vi "Configure.vi"(8 "error in (no error)":errorcluster, 11 "ImageStack in":refnum<class "ImageStack.lvclass">) -> (0 "error out":errorcluster, 2 "cancelled?":bool, 3 "ImageStack out":refnum<class "ImageStack.lvclass">)   [LabVIEW 2012, in "ImageStack.lvclass"]
doc: "The configure method configures the details for the RabbitMQ connection. \n\nIn the derived class, make a call to the parent for setting these parameters."
uses:
  ImageStack.lvclass
  <vilib>/Utility/miscctls.llb/LVPointTypeDef.ctl
  ImageStack.lvclass/ImageStack.ctl
  <vilib>/Distrio/Murmex/Murmex/Murmex.lvclass
panel:
  in  "AOTF component name":string
  in  "button:cancel":bool
  in  "button:configure murmex":bool
  in  "button:ok":bool
  in  "Stages component name":string
  in  "Camera component name":string
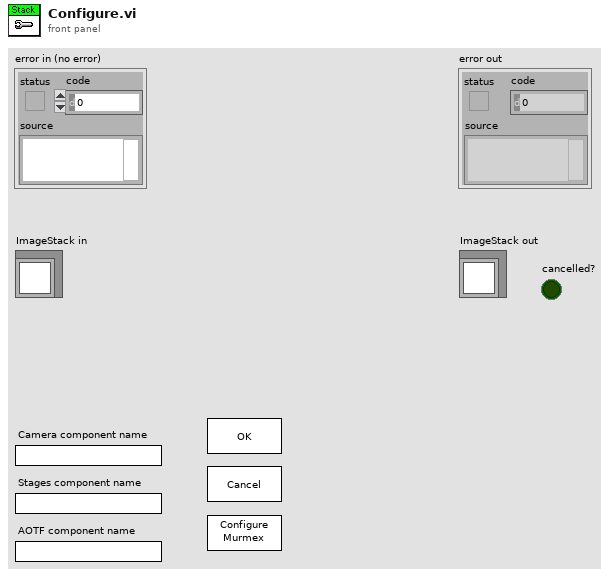
[diagram p1: front panel]
types:
  T1 = typedef "LVPointTypeDef.ctl" = cluster{"Horizontal":i16, "Vertical":i16}
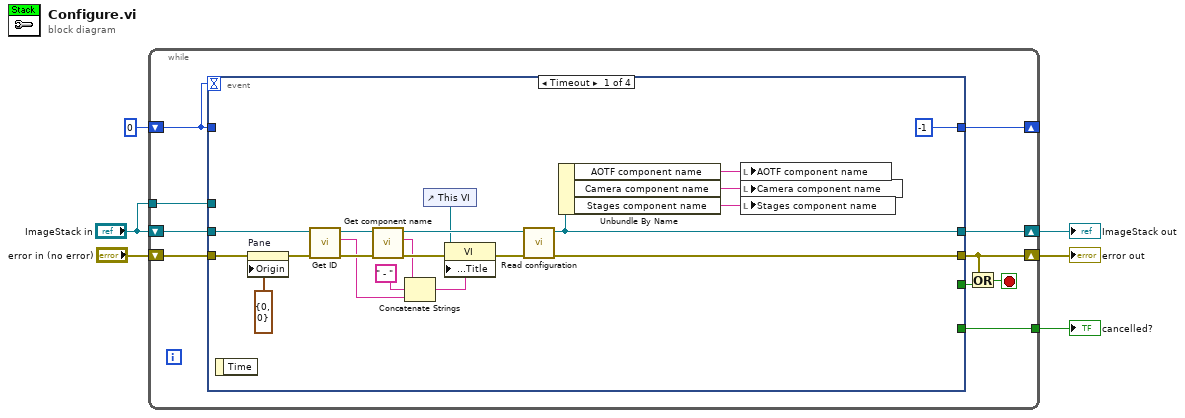
[diagram p0: block diagram]
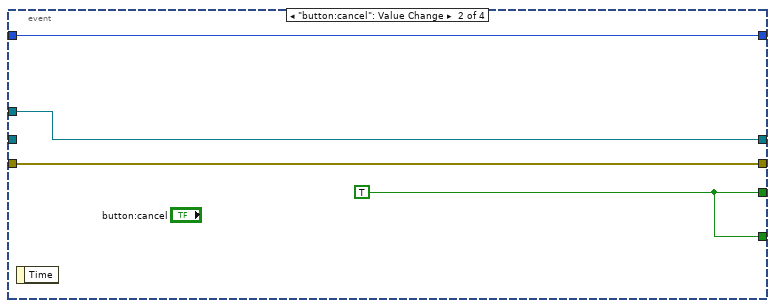
[diagram p2: hidden frame]
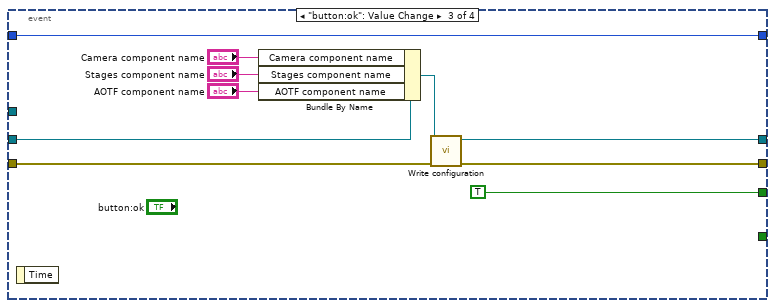
[diagram p3: hidden frame]
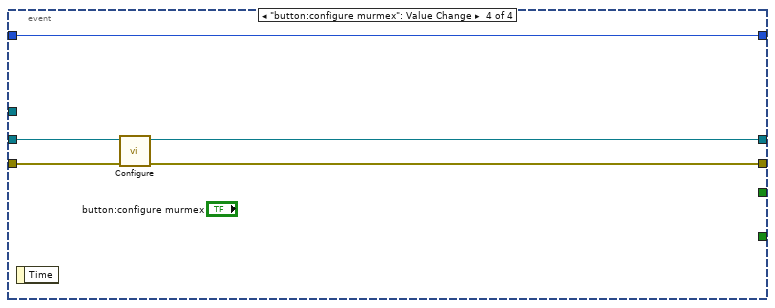
[diagram p4: hidden frame]
diagram:
  n1 = while {
    shift-right: [w11] -> w1
    shift-left: "ImageStack in" -> [w12]
    shift-right: [w13] -> w2
    shift-left: "error in (no error)" -> [w15]
    shift-right: [w16] -> _
    shift-left: 0 -> [w8]
    tunnel: "ImageStack in" -> [w9]
    tunnel: [w7] -> w3
    stop <- w14 stop-if-true
    n2 = event shown="[0] Timeout" {
      selector: _ -> [_ _ _ _]
      dyn-events: _ -> [_ _ _ _]
      timeout: w8 -> [_ _ _ _]
      tunnel: [-1 w38 w42 w51] -> w16
      tunnel: w15 -> [w34 w40 w46 w54]
      tunnel: [w35 w40 w44 w52] -> w13
      tunnel: w12 -> [w31 _ w50 w55]
      tunnel: [w20 w39 w45 w53] -> w11
      tunnel: [_ w37 TRUE _] -> w10
      tunnel: w9 -> [_ w39 _ _]
      tunnel: w8 -> [_ w38 w42 w51]
      tunnel: [_ w37 _ _] -> w7
      event Timeout {
        n3 = event-data() -> ()  [unwired: 1 in, 1 out]
        n4 = property on="Pane" class="Pane"(error in=w34, "Origin"=T1 {"Horizontal"=0, "Vertical"=0}) -> (error out=w32:errorcluster)  [unwired: 1 in, 1 out]
        n5 = call <vilib>:"Get ID.vi"("error in (no error)"=w32, "Murmex in"=w31) -> ("error out"=w29:errorcluster, "component id"=w25:string, "Murmex out"=w30:refnum<class "ImageStack.lvclass">)  [unwired: 7 in]
        n6 = call <vilib>:"Get component name.vi"("error in (no error)"=w29, "Murmex in"=w30) -> ("error out"=w28:errorcluster, "component name"=w26:string, "Murmex out"=w27:refnum<class "ImageStack.lvclass">)  [unwired: 7 in]
        n7 = Concatenate Strings(w26, " - " ("element"), w25) -> (w21:string)
        n8 = control-ref of="This VI"() -> (w22:refnum<vi>)
        n9 = property class="VI"(reference=w22, error in=w28, "Front Panel.Title"=w21) -> (error out=w23:errorcluster)  [unwired: 1 out]
        n10 = call <vilib>:"Read configuration.vi"("error in (no error)"=w23, "Murmex in"=w27) -> ("error out"=w35:errorcluster, "Murmex out"=w20:refnum<class "ImageStack.lvclass">)  [unwired: 7 in, 1 out]
        n11 = Unbundle By Name(w20) -> ("AOTF component name"=w17:string, "Camera component name"=w19:string, "Stages component name"=w18:string)
        n12 = local write "AOTF component name"(w17) -> ()
        n13 = local write "Camera component name"(w19) -> ()
        n14 = local write "Stages component name"(w18) -> ()
      }
      event "button:cancel": Value Change {
        w37 = TRUE
        n15 = event-data() -> ()  [unwired: 1 in, 1 out]
      }
      event "button:ok": Value Change {
        n16 = event-data() -> ()  [unwired: 1 in, 1 out]
        n17 = Bundle By Name(cluster=w50, "Camera component name"="Camera component name", "Stages component name"="Stages component name", "AOTF component name"="AOTF component name") -> (w49:refnum<class "ImageStack.lvclass">)
        n18 = call <vilib>:"Write configuration.vi"("error in (no error)"=w46, "Murmex in"=w49) -> ("error out"=w44:errorcluster, "Murmex out"=w45:refnum<class "ImageStack.lvclass">)  [unwired: 8 in]
      }
      event "button:configure murmex": Value Change {
        n19 = event-data() -> ()  [unwired: 1 in, 1 out]
        n20 = call-parent "Configure.vi"("error in (no error)"=w54, "Murmex in"=w55) -> ("error out"=w52:errorcluster, "Murmex out"=w53:refnum<class "ImageStack.lvclass">)  [unwired: 7 in, 1 out]
      }
    }
    n21 = Or(x=w13, y=w10) -> (x .or. y?=w14:bool)
  }
  "error out" <- w2
  "ImageStack out" <- w1
  "cancelled?" <- w3
